vi "Dbl_to_8bit.vi"(11 "Numeric in":dbl) -> (3 "Numeric out":u8)   [LabVIEW 2013]
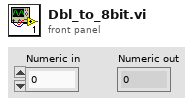
[diagram p1: front panel]
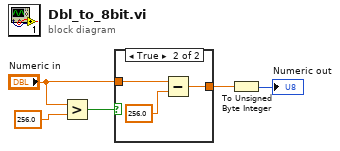
[diagram p0: block diagram]
diagram:
  n1 = Greater?(x="Numeric in", y=256.0) -> (0:w3:bool)
  n2 = case shown="True" w3 {
    tunnel: "Numeric in" -> [w6 w8]
    tunnel: [w6 w7] -> w5
    frame False {
    }
    frame True {
      n3 = Subtract(x=w8, y=256.0) -> (x-y=w7:dbl)
    }
  }
  n4 = To Unsigned Byte Integer(number=w5) -> (unsigned 8bit integer=→"Numeric out":u8)
